vi "setSettingDirectory.vi"(10 "SettingDirectory":path, 11 "BaseSetting in":refnum<class "Setting.lvclass">) -> (3 "BaseSetting out":refnum<class "Setting.lvclass">)   [LabVIEW 2016, in "Settings.lvlib" / "Setting.lvclass"]
uses:
  Setting.lvclass
  Setting.lvclass/Setting.ctl
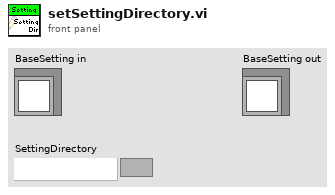
[diagram p1: front panel]
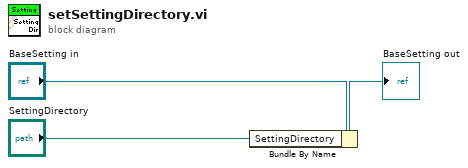
[diagram p0: block diagram]
diagram:
  n1 = Bundle By Name(cluster="BaseSetting in", "SettingDirectory"="SettingDirectory") -> (→"BaseSetting out":refnum<class "Setting.lvclass">)
